vi "PH_Timing.set BNC Channel Defaults.vi"(0 "i ref in":refnum<vi>, 1 "Instancename":string="N/A", 2 "Channel":i32(ring)=1 items=["System (To)", "Channel A", "Channel B", "Channel C", "Channel D", "Channel E", "Channel F", "Channel G", "Channel H"], 5 "error in (no error)":errorcluster) -> (14 "i ref out":refnum<vi>, 19 "error out":errorcluster)   [LabVIEW 2014, in "PH_Timing.lvlib"]
doc: "By this VI the default settings of a BNC 555 generator channel are set to be:\n\nGate enabled = false\nChannel Mode = Single Shot"
uses:
  PH_Timing.lvlib
  CSDigitalIO/BNC555/BNC555.lvlib
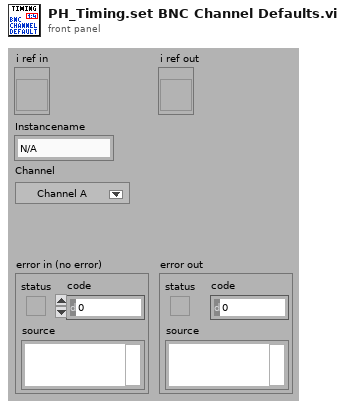
[diagram p1: front panel]
types:
  T1 = enum16{"Normal", "Single", "Burst", "Divide by N"}
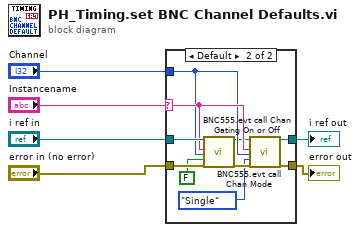
[diagram p0: block diagram]
diagram:
  n1 = case shown="Default" "Instancename" {
    selector: "Instancename" -> [_ w16]
    tunnel: "Channel" -> [_ w13]
    tunnel: "error in (no error)" -> [w7 w18]
    tunnel: "i ref in" -> [w8 w17]
    tunnel: [w8 w15] -> w4
    tunnel: [w7 w14] -> w3
    frame "", "N/A" {
    }
    frame Default {
      n2 = call "BNC555.evt call Chan Gating On or Off.vi"("i ref in"=w17, "Generator Instance"=w16, "Channel"=w13, "Gating State"=FALSE ("Gate enabled (false)"), "error in (no error)"=w18) -> ("i ref out"=w12:refnum<vi>, "error out"=w11:errorcluster)  [unwired: 13 in]
      n3 = call "BNC555.evt call Chan Mode.vi"("i ref in"=w12, "Generator Instance"=w16, "Channel"=w13, "Mode"=T1."Single" ("Mode (0:Normal)"), "error in (no error)"=w11) -> ("i ref out"=w15:refnum<vi>, "error out"=w14:errorcluster)  [unwired: 13 in]
    }
  }
  "i ref out" <- w4
  "error out" <- w3
